vi "Defocus and Spherical Comp V2.vi"(1 "Spherical Step":dbl, 2 "Defocus Step":dbl, 3 "Step #":i32) -> ()   [LabVIEW 2014]
uses:
  DM_Dual_V2/Controls/Standard Action.ctl
panel:
  out "Map 2":dbl[][](graph)
  out "map 1":dbl[][](graph)
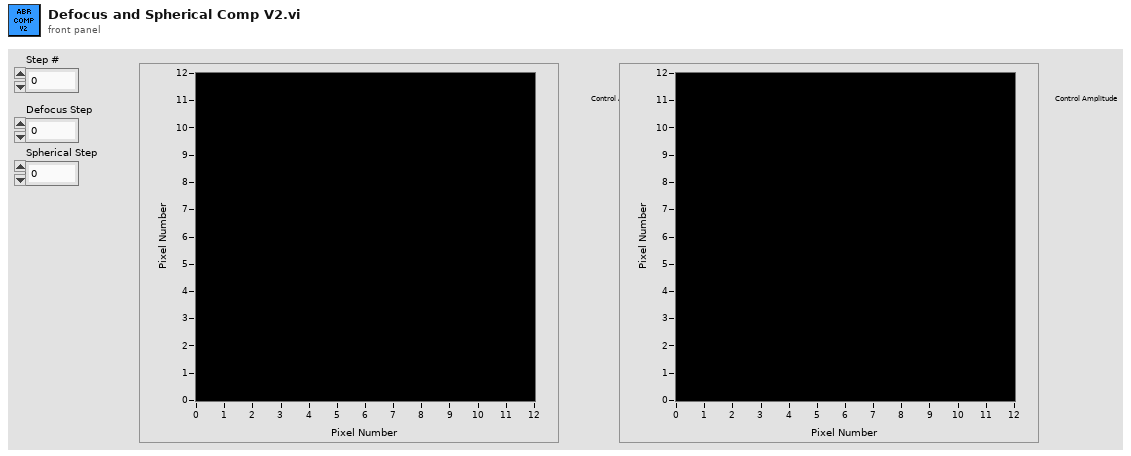
[diagram p1: front panel]
types:
  T1 = typedef "Standard Action.ctl" = enum16{"Read", "Write"}
  T2 = typedef "MirrorModes_DUAL.ctl" = cluster{"Mode":string, "Amplitude":dbl}[][]
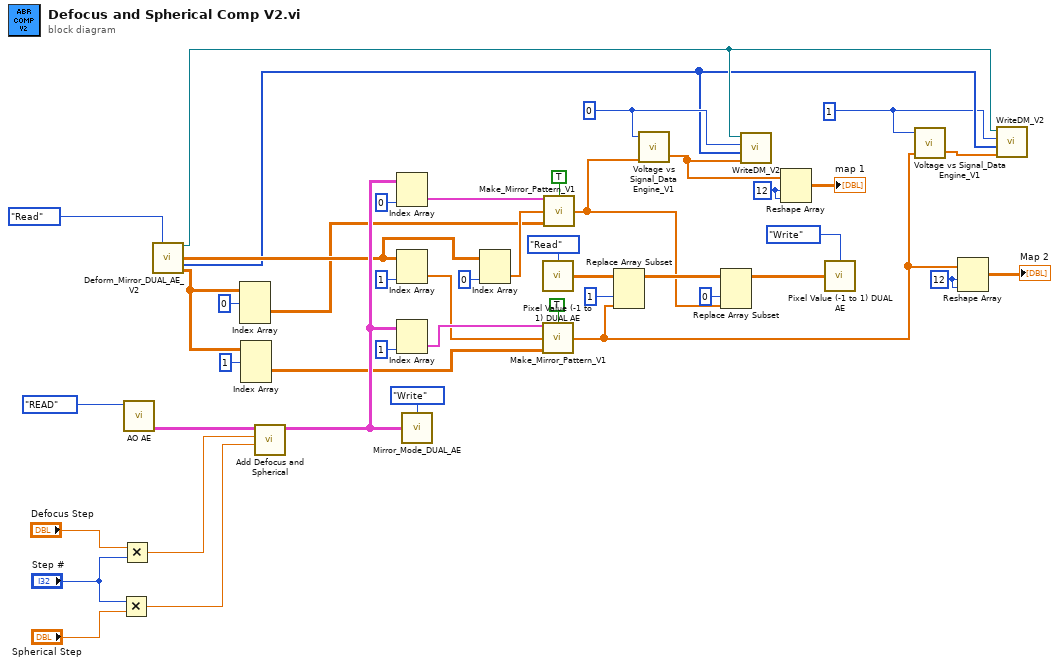
[diagram p0: block diagram]
diagram:
  w11 = 12 ("dimension size")
  w14 = 12 ("dimension size")
  w28 = 1 ("disabled index (col)")
  w32 = 0 ("disabled index (col)")
  n1 = Multiply(x="Step #", y="Spherical Step") -> (x*y=w23:dbl)
  n2 = Multiply(x="Defocus Step", y="Step #") -> (x*y=w24:dbl)
  n3 = call "AO AE.vi"("Action"=enum16{"READ", "WRITE"}."READ") -> ("Mirror Modes Out"=w6:T2)  [unwired: 8 in, 2 out]
  n4 = call "Deform_Mirror_DUAL_AE_V2.vi"("Action"=Standard_Action."Read") -> ("Refnum Out"=w30:refnum<k7>, "Flat Files Out"=w40:dbl[][], "Multi Map Data Out"=w29:i32[], "Mode Matrix Out"=w3:dbl[][][])  [unwired: 10 in, 1 out]
  n5 = Index Array(array=w3, index (dim 0)=0 ("index (page)")) -> (element=w4:dbl[][])  [unwired: 2 in]
  n6 = Index Array(array=w3, index (dim 0)=1 ("index (page)")) -> (element=w1:dbl[][])  [unwired: 2 in]
  n7 = call "Add Defocus and Spherical.vi"("Spherical Comp"=w23, "Defocus Comp"=w24, "Mirror Modes in"=w6) -> ("Mirror Modes out"=w43:T2)  [unwired: 8 in]
  n8 = Index Array(array=w43, index (col)=0 ("disabled index (col)")) -> (element=w34:cluster{"Mode":string, "Amplitude":dbl}[])  [unwired: 1 in]
  n9 = Index Array(array=w40, index (col)=1 ("disabled index (col)")) -> (element=w36:dbl[])  [unwired: 1 in]
  n10 = Index Array(array=w43, index (col)=1 ("disabled index (col)")) -> (element=w38:cluster{"Mode":string, "Amplitude":dbl}[])  [unwired: 1 in]
  n11 = call "Mirror_Mode_DUAL_AE.vi"("Action"=Standard_Action."Write", "Mirror Modes In"=w43) -> ()  [unwired: 13 in, 1 out]
  n12 = Index Array(array=w40, index (col)=0 ("disabled index (col)")) -> (element=w33:dbl[])  [unwired: 1 in]
  n13 = call "Pixel Value (-1 to 1) DUAL AE.vi"("Action"=Standard_Action."Read") -> ("Pixel Value (-1 to 1) Out"=w20:dbl[][])  [unwired: 14 in]
  n14 = call "Make_Mirror_Pattern_V1.vi"("Mirror Modes In"=w38, "Flat On?"=TRUE, "Flat File In"=w36, "Mirror Modes Array"=w1) -> ("Pixel Value U (-1 to 1)"=w10:dbl[])  [unwired: 11 in]
  n15 = call "Make_Mirror_Pattern_V1.vi"("Mirror Modes In"=w34, "Flat On?"=TRUE, "Flat File In"=w33, "Mirror Modes Array"=w4) -> ("Pixel Value U (-1 to 1)"=w16:dbl[])  [unwired: 11 in]
  n16 = Replace Array Subset(array=w20, new element=w10, index (col)=1 ("disabled index (col)")) -> (w18:dbl[][])  [unwired: 1 in]
  n17 = call "Voltage vs Signal_Data Engine_V1.vi"("Control Signal In (-1~1)"=w16, "DM #"=w32) -> ("Voltage Out (0~Max. Vol.)"=w13:dbl[])  [unwired: 1 in, 1 out]
  n18 = Replace Array Subset(array=w18, new element=w16, index (col)=0 ("disabled index (col)")) -> (w15:dbl[][])  [unwired: 1 in]
  n19 = call "WriteDM_V2.vi"("reference in"=w30, "nDevId"=w32, "MultiDM  Mapping"=w29, "Voltage Array in"=w13) -> ()  [unwired: 2 in, 2 out]
  n20 = Reshape Array(w13, w14, w14) -> (→"map 1":dbl[][])
  n21 = call "Pixel Value (-1 to 1) DUAL AE.vi"("Action"=Standard_Action."Write", "Pixel Value (-1 to 1)"=w15) -> ()  [unwired: 13 in, 1 out]
  n22 = call "Voltage vs Signal_Data Engine_V1.vi"("Control Signal In (-1~1)"=w10, "DM #"=w28) -> ("Voltage Out (0~Max. Vol.)"=w31:dbl[])  [unwired: 1 in, 1 out]
  n23 = Reshape Array(w10, w11, w11) -> (→"Map 2":dbl[][])
  n24 = call "WriteDM_V2.vi"("reference in"=w30, "nDevId"=w28, "MultiDM  Mapping"=w29, "Voltage Array in"=w31) -> ()  [unwired: 2 in, 2 out]
